vi "Update Car Wash Indicators.vi"(8 "error in (no error)":errorcluster, 10 "Car Wash Indicators":T1, 11 "Simulated Wash Display Console Actor in":refnum<class "Simulated Wash Display Console Actor.lvclass">) -> (0 "error out":errorcluster, 3 "Simulated Wash Display Console Actor out":refnum<class "Simulated Wash Display Console Actor.lvclass">)   [LabVIEW 2019, in "Simulated Wash Display Console Actor.lvlib" / "Simulated Wash Display Console Actor.lvclass"]
uses:
  Simulated Wash Display Console Actor.lvclass
  Sim Entry Console Actor/Sim Entry Console Actor/Wash steps selection -Buttons.ctl
  Simulated Wash Display Console Actor.lvclass/Simulated Wash Display Console Actor.ctl
  Sim Entry Console Actor/Sim Entry Console Actor/Simulated Entry Console Actor.lvclass
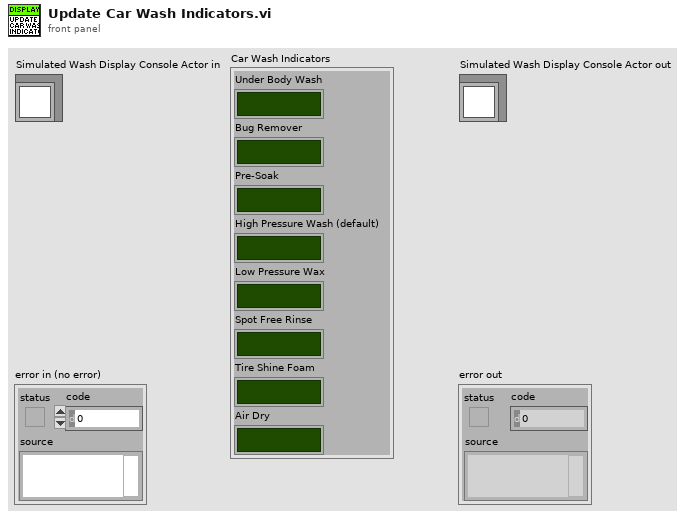
[diagram p1: front panel]
types:
  T1 = typedef "Simulated Entry Console Actor.lvlib/Simulated Entry Console Actor.lvclass/Wash steps selection -Buttons.ctl" = cluster{"Under Body Wash":bool, "Bug Remover":bool, "Pre-Soak":bool, "High Pressure Wash (default)":bool, "Low Pressure Wax":bool, "Spot Free Rinse":bool, "Tire Shine Foam":bool, "Air Dry":bool}
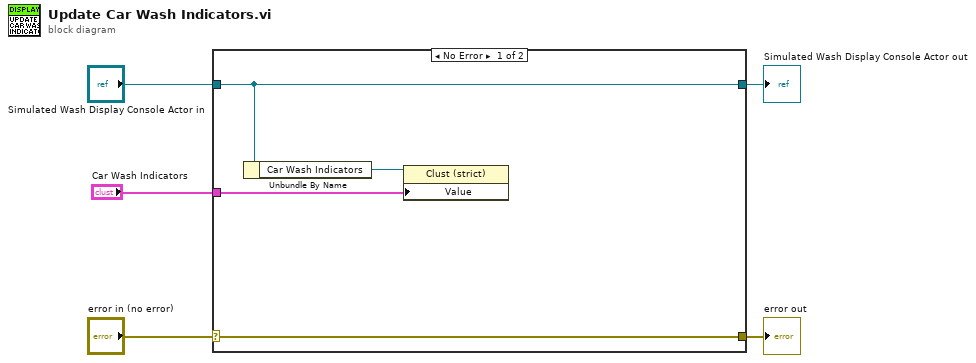
[diagram p0: block diagram]
diagram:
  n1 = case shown="No Error" "error in (no error)" {
    selector: "error in (no error)" -> [w9 w10]
    tunnel: [w9 w10] -> w4
    tunnel: [w7 w11] -> w2
    tunnel: "Simulated Wash Display Console Actor in" -> [w7 w11]
    tunnel: "Car Wash Indicators" -> [w6 _]
    frame No Error {
      n2 = Unbundle By Name(w7) -> ("Car Wash Indicators"=w8:refnum<vi>)
      n3 = property class="Clust (strict)"(reference=w8, "Value"=w6) -> ()  [unwired: 1 in, 2 out]
    }
    frame Error {
    }
  }
  "error out" <- w4
  "Simulated Wash Display Console Actor out" <- w2
